vi "AppLauncher.vi"() -> ()   [LabVIEW 2016, in "Instrument.Oxford1820.lvclass"]
uses:
  Instrument.Oxford1820.lvclass
  <vilib>/JKI/JKI SMO/SMO/SMO.lvclass
  <vilib>/JKI/JKI SMO/SMO/Typedefs/SMOState --Enum.ctl
  <vilib>/JKI/JKI SMO/SMO.UI/SMO.UI.lvclass
  Instrument.Oxford1820 UI/Instrument.Oxford1820 UI.lvclass
  <vilib>/Utility/sysdir.llb/System Directory Type.ctl
  <userlib>/LevyLab/Levylab Instruments/SMOs/Instrument/Instrument.lvclass
  C:/Program Files (x86)/National Instruments/LabVIEW 2016/vi.lib/JKI/JKI SMO/SMO/SMO.lvclass
  C:/Program Files (x86)/National Instruments/LabVIEW 2016/user.lib/LevyLab/Levylab Instruments/SMOs/Instrument/Instrument.lvclass
  C:/Program Files (x86)/National Instruments/LabVIEW 2016/vi.lib/JKI/JKI SMO/SMO.UI/SMO.UI.lvclass
panel:
  out "Hardware Address":string
  out "UI SMO State":T1
  out "SMO State":T1
  out "error out":errorcluster
  in  "Stop":bool
  # "Instrument.SR7270 SMO Launcher"
  # "For instructions on how to use the JKI State Machine Objects, examples and video tutorials, visit:\nhttp://jki.net/state-machine-objects/\n\nJKI State Machine Objects™\nhttp://jki.net/state-machine-objects/\nCopyright (C) 2005-2015, JKI <info@jki.net>\nALL RIGHTS RESERVED"
  # "Starting Example Instrument..."
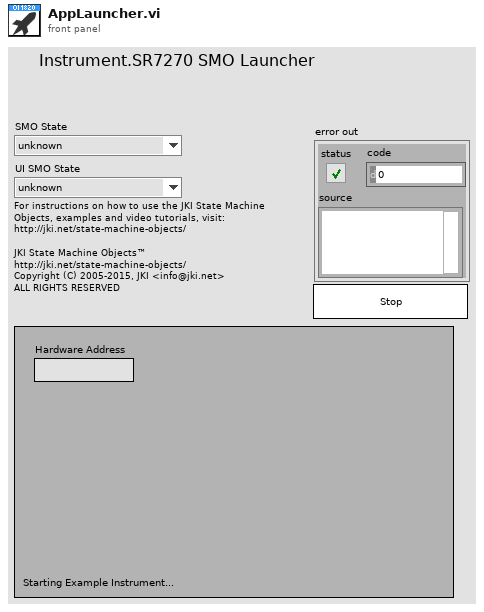
[diagram p1: front panel]
types:
  T1 = typedef "SMO.lvclass/SMOState --Enum.ctl" = enum16{"unknown", "Created", "Started", "Stopped"}
  T2 = typedef "System Directory Type.ctl" = i32
  T3 = typedef "SMO.lvclass/Public Events.ctl" = cluster{"Error":refnum<user-event>, "State":refnum<user-event>, "Reserve State":refnum<user-event>}
  T4 = cluster{"Event Registration Refnum":refnum<event-registration>, "Event Registration Refnum":refnum<event-registration>}
  T5 = enum32{"Invalid", "Standard", "Closed", "Hidden", "Minimized", "Maximized"}
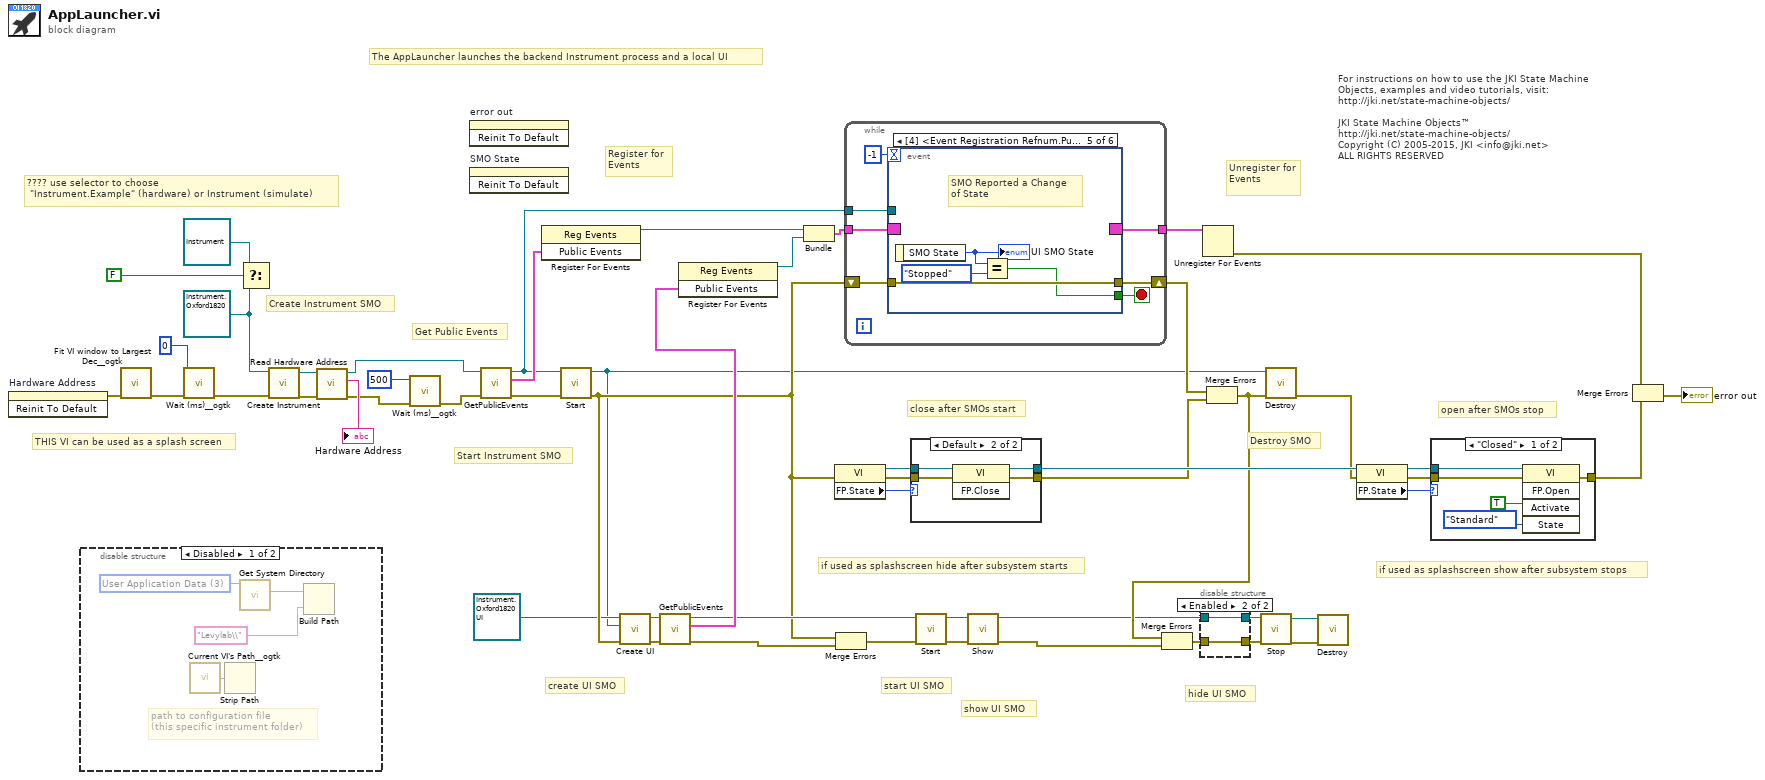
[diagram p0: block diagram]
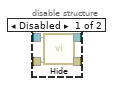
[diagram p2: hidden frame]
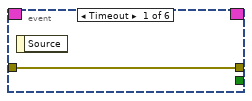
[diagram p5: hidden frame]
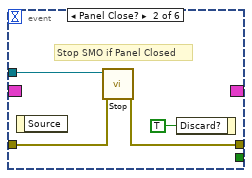
[diagram p6: hidden frame]
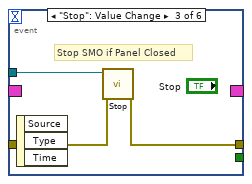
[diagram p7: hidden frame]
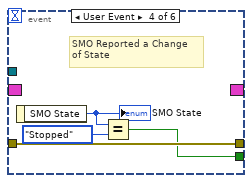
[diagram p8: hidden frame]
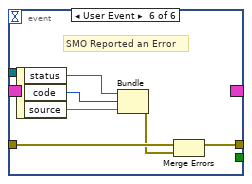
[diagram p9: hidden frame]
diagram:
  w7 = refnum<class "Instrument.Oxford1820.lvclass"> refnum ("Instrument.SR7270.lvclass")
  # "???? use selector to choose\n \"Instrument.Example\" (hardware) or Instrument (simulate)"
  # "open after SMOs stop"
  # "close after SMOs start"
  # "hide UI SMO"
  # "show UI SMO"
  # "start UI SMO"
  # "create UI SMO"
  # "if used as splashscreen show after subsystem stops"
  # "if used as splashscreen hide after subsystem starts"
  # "THIS VI can be used as a splash screen"
  # "The AppLauncher launches the backend Instrument process and a local UI"
  # "Get Public Events"
  # "Start Instrument SMO"
  # "Destroy SMO"
  # "Create Instrument SMO"
  # "Unregister for Events"
  # "Register for Events"
  # "For instructions on how to use the JKI State Machine Objects, examples and video tutorials, visit:\nhttp://jki.net/state-machine-objects/\n\nJKI State Machine Objects™\nhttp://jki.net/state-machine-objects/\nCopyright (C) 2005-2015, JKI <info@jki.net>\nALL RIGHTS RESERVED"
  n1 = invoke on="Hardware Address" class="Str" method="Reinit To Default"() -> (error out=w11:errorcluster)  [unwired: 3 in, 2 out]
  n2 = disable-structure shown="Disabled" {
    frame Disabled {
      w56 = T2 3 items=["User Home"=0, "User Desktop"=1, "User Documents"=2, "User Application Data"=3, "User Preferences"=4, "User Temporary"=5, "Public Documents"=6, "Public Application Data"=7, "Public Preferences"=8, "Public Cache"=13, "System Core Libraries"=9, "System Installed Libraries"=10, "Application Files"=11, "Boot Volume Root"=12] ("system directory type")
      # "path to configuration file\n(this specific instrument folder)"
      n3 = call <userlib>:"Current VI's Path__ogtk.vi"() -> ("Current VI's Path (+ Relative)"=w57:path)  [unwired: 1 in]
      n4 = Strip Path(path=w57) -> ()  [unwired: 2 out]
      n5 = call <vilib>:"Get System Directory.vi"("system directory type"=w56) -> ("system directory"=w55:path)  [unwired: 10 in]
      n6 = Build Path(base path=w55, name or relative path="Levylab\\") -> ()  [unwired: 1 out]
    }
    frame Enabled {
    }
  }
  n7 = call <userlib>:"Fit VI window to Largest Dec__ogtk.vi"("error in (no error)"=w11) -> ("error out"=w42:errorcluster)  [unwired: 5 in, 1 out]
  n8 = call <userlib>:"Wait (ms)__ogtk.vi"("error in (no error)"=w42, "milliseconds to wait"=u32 0) -> ("error out"=w8:errorcluster)  [unwired: 8 in, 1 out]
  n9 = Select(t=refnum<class "Instrument.lvclass"> refnum ("Instrument.lvclass"), s=FALSE, f=w7) -> ()  [unwired: 1 out]
  n10 = call-dynamic "Create Instrument.vi"("error in (no error)"=w8, "Instrument in"=w7) -> ("error out"=w16:errorcluster, "Instrument out"=w13:refnum<class "Instrument.Oxford1820.lvclass">)  [unwired: 8 in]
  n11 = call-dynamic "Read Hardware Address.vi"("error in (no error)"=w16, "Instrument in"=w13) -> ("error out"=w15:errorcluster, "Hardware Address"=→"Hardware Address":string, "Instrument out"=w6:refnum<class "Instrument.Oxford1820.lvclass">)  [unwired: 7 in]
  n12 = call <userlib>:"Wait (ms)__ogtk.vi"("error in (no error)"=w15, "milliseconds to wait"=u32 500) -> ("error out"=w12:errorcluster)  [unwired: 8 in, 1 out]
  n13 = invoke on="error out" class="Clust (strict)" method="Reinit To Default"() -> ()  [unwired: 3 in, 3 out]
  n14 = invoke on="SMO State" class="Enum (strict)" method="Reinit To Default"() -> ()  [unwired: 3 in, 3 out]
  n15 = call <vilib>:"GetPublicEvents.vi"("error in (no error)"=w12, "SMO"=w6) -> ("error out"=w48:errorcluster, "Public Events"=w50:T3, "SMO out"=w49:refnum<class "Instrument.Oxford1820.lvclass">)  [unwired: 7 in]
  n16 = register-events(w50) -> (reference out=w41:refnum<event-registration>)  [unwired: 2 in, 1 out]
  n17 = call <vilib>:"Start.vi"("error in (no error)"=w48, "SMO"=w49) -> ("error out"=w5:errorcluster, "SMO out"=w1:refnum<class "Instrument.Oxford1820.lvclass">)  [unwired: 8 in]
  n18 = call "Create UI.vi"("error in (no error)"=w5, "Instrument.Oxford1820 in"=w1, "Instrument.Oxford1820 UI in"=refnum<class "Instrument.Oxford1820 UI.lvclass"> refnum ("SR7220 UI.lvclass")) -> ("error out"=w2:errorcluster, "Instrument.Oxford1820 UI out"=w3:refnum<class "Instrument.Oxford1820 UI.lvclass">)  [unwired: 7 in]
  n19 = call <vilib>:"GetPublicEvents.vi"("error in (no error)"=w2, "SMO"=w3) -> ("error out"=w32:errorcluster, "Public Events"=w38:T3, "SMO out"=w33:refnum<class "Instrument.Oxford1820 UI.lvclass">)  [unwired: 7 in]
  n20 = register-events(w38) -> (reference out=w39:refnum<event-registration>)  [unwired: 2 in, 1 out]
  n21 = Bundle("Event Registration Refnum"=w41, "Event Registration Refnum"=w39) -> (w40:T4)  [unwired: 1 in]
  n22 = property class="VI"(error in=w5) -> (reference out=w22:refnum<vi>, error out=w23:errorcluster, "FP.State"=w21:T5)  [unwired: 1 in]
  n23 = Merge Errors(w5, w32) -> (w37:errorcluster)
  n24 = while {
    shift-right: [w63] -> w47
    shift-left: w5 -> [w62]
    tunnel: w40 -> [w61]
    tunnel: [w60] -> w53
    tunnel: w49 -> [w59]
    stop <- w64 stop-if-true
    n25 = event shown="[4] <Event Registration Refnum.Public Events.State>: User Event" {
      selector: w61 -> [_ _ _ _ _ _]
      dyn-events: [_ _ _ _ _ _] -> w60
      timeout: -1 -> [_ _ _ _ _ _]
      tunnel: [_ _ _ w73 w77 _] -> w64
      tunnel: w59 -> [_ w69 w72 _ _ _]
      tunnel: [w65 w68 w71 w76 w80 w84] -> w63
      tunnel: w62 -> [w65 w67 w70 w76 w80 w82]
      event Timeout {
        n26 = event-data() -> ()  [unwired: 1 in, 1 out]
      }
      event Panel Close? {
        # "Stop SMO if Panel Closed"
        n27 = event-data() -> ()  [unwired: 1 in, 1 out]
        n28 = call <vilib>:"Stop.vi"("error in (no error)"=w67, "SMO"=w69) -> ("error out"=w68:errorcluster)  [unwired: 8 in, 1 out]
        n29 = event-data("Discard?"=TRUE ("OK")) -> ()  [unwired: 1 in, 1 out]
      }
      event "Stop": Value Change {
        # "Stop SMO if Panel Closed"
        n30 = event-data() -> ()  [unwired: 1 in, 3 out]
        n31 = call <vilib>:"Stop.vi"("error in (no error)"=w70, "SMO"=w72) -> ("error out"=w71:errorcluster)  [unwired: 8 in, 1 out]
      }
      event User Event {
        # "SMO Reported a Change\nof State"
        n32 = event-data() -> ("SMO State"=w75:T1)  [unwired: 1 in]
        "SMO State" <- w75
        n33 = Equal?(x=w75, y=SMOState_--Enum."Stopped") -> (x = y?=w73:bool)
      }
      event User Event {
        # "SMO Reported a Change\nof State"
        n34 = event-data() -> ("SMO State"=w79:T1)  [unwired: 1 in]
        "UI SMO State" <- w79
        n35 = Equal?(x=w79, y=SMOState_--Enum."Stopped") -> (x = y?=w77:bool)
      }
      event User Event {
        # "SMO Reported an Error"
        n36 = event-data() -> ("status"=w83:bool, "code"=w86:i32, "source"=w85:string)  [unwired: 1 in]
        n37 = Bundle("status"=w83, "code"=w86, "source"=w85) -> (w81:errorcluster)  [unwired: 1 in]
        n38 = Merge Errors(w82, w81) -> (w84:errorcluster)
      }
    }
  }
  n39 = case shown="Default" w21 {
    tunnel: [w88 w92] -> w43
    tunnel: w23 -> [w88 w91]
    tunnel: w22 -> [w87 w90]
    tunnel: [w87 w89] -> w46
    frame "Invalid", "Closed" {
    }
    frame Default {
      n40 = invoke class="VI" method="FP.Close"(reference=w90, error in=w91) -> (reference out=w89:refnum<vi>, error out=w92:errorcluster)  [unwired: 1 in, 1 out]
    }
  }
  n41 = call <vilib>:"Start.vi"("error in (no error)"=w37, "SMO"=w33) -> ("error out"=w31:errorcluster, "SMO out"=w30:refnum<class "Instrument.Oxford1820 UI.lvclass">)  [unwired: 8 in]
  n42 = call <vilib>:"Show.vi"("error in (no error)"=w31, "SMO.UI"=w30) -> ("error out"=w29:errorcluster, "SMO.UI out"=w25:refnum<class "Instrument.Oxford1820 UI.lvclass">)  [unwired: 8 in]
  n43 = Unregister For Events(event registration refnum=w53) -> (error out=w52:errorcluster)  [unwired: 1 in]
  n44 = Merge Errors(w47, w43) -> (w34:errorcluster)
  n45 = Merge Errors(w34, w29) -> (w26:errorcluster)
  n46 = disable-structure shown="Enabled" {
    disable-tunnel: [w96 w97] -> w28
    disable-tunnel: [w95 w98] -> w27
    disable-tunnel: w26 -> [w94 w97]
    disable-tunnel: w25 -> [w93 w98]
    frame Disabled {
      n47 = call <vilib>:"Hide.vi"("error in (no error)"=w94, "SMO.UI"=w93) -> ("error out"=w96:errorcluster, "SMO.UI out"=w95:refnum<class "Instrument.Oxford1820 UI.lvclass">)  [unwired: 8 in]
    }
    frame Enabled {
    }
  }
  n48 = call <vilib>:"Stop.vi"("error in (no error)"=w28, "SMO"=w27) -> ("error out"=w36:errorcluster, "SMO out"=w35:refnum<class "Instrument.Oxford1820 UI.lvclass">)  [unwired: 8 in]
  n49 = call <vilib>:"Destroy.vi"("error in (no error)"=w34, "SMO"=w1) -> ("error out"=w45:errorcluster)  [unwired: 9 in]
  n50 = call <vilib>:"Destroy.vi"("error in (no error)"=w36, "SMO"=w35) -> ()  [unwired: 9 in, 1 out]
  n51 = property class="VI"(reference=w46, error in=w45) -> (reference out=w19:refnum<vi>, error out=w20:errorcluster, "FP.State"=w18:T5)
  n52 = case shown="\"Closed\"" w18 {
    tunnel: [w101 w104] -> w44
    tunnel: w20 -> [w100 w104]
    tunnel: w19 -> [w99 _]
    frame "Closed" {
      n53 = invoke class="VI" method="FP.Open"(reference=w99, error in=w100, "Activate"=TRUE, "State"=T5."Standard") -> (error out=w101:errorcluster)  [unwired: 1 in, 4 out]
    }
    frame Default {
    }
  }
  n54 = Merge Errors(w52, w44) -> (→"error out":errorcluster)
